vi "Autonomous Independent.vi"() -> ()   [LabVIEW 2013]
doc: "This VI is called when autonomous begins, and will automatically be terminated when autonomous ends. You can carry out timed or sensor driven robot movement independently without needing to return to the caller."
uses:
  Robot Global Data.vi
  <vilib>/Rock Robotics/WPI/RobotDrive/WPI_RobotDriveArcadeDrive_Standard(NoSaturation).vi
  <vilib>/Rock Robotics/WPI/RobotDrive/WPI_RobotDriveGetSetRefNum.vi
  <vilib>/Rock Robotics/WPI/Joystick/WPI_JoystickGetSetRefNum.vi
panel:
  out "Current Movement, for debugging":T1 {"Y Joystick Value" scale=1.0..-1.0; "X Joystick Value" scale=-1.0..1.0}
  in  "Array of robot movements":T2(array[cluster]) {"Y Joystick Value" scale=1.0..-1.0; "X Joystick Value" scale=-1.0..1.0}
  # "Be sure to right-click and choose Data Operations>>Make Current Value default if you want to save the array values with the VI"
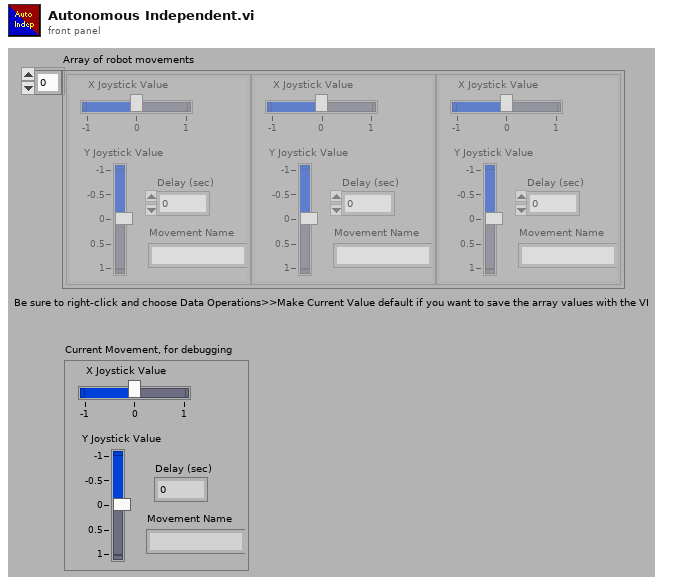
[diagram p1: front panel]
types:
  T1 = cluster{"X Joystick Value":dbl, "Y Joystick Value":dbl, "Delay (sec)":dbl, "Movement Name":string}
  T2 = cluster{"X Joystick Value":dbl, "Y Joystick Value":dbl, "Delay (sec)":dbl, "Movement Name":string}[]
  T3 = typedef "WPI_JoystickDevRef.ctl" = cluster{"Device":T4}
  T4 = typedef "WPI_JoystickDeviceEnum.ctl" = enum16{"USB 1", "USB 2", "USB 3", "USB 4", "Kinect 1", "Kinect 2"}
  T5 = cluster{"axis 1 (x)":dbl, "axis 2 (y)":dbl, "axis 3 (throttle)":dbl, "axis 4":dbl, "axis 5":dbl, "axis 6":dbl}
  T6 = typedef "WPI_RobotDriveDevRef.ctl" = cluster{"DevStatus":errorcluster, "Motors[]":T7[], "Square Inputs":bool, "Max Output":dbl, "Isochronous":bool}
  T7 = typedef "WPI_MotorControlDeviceRef.ctl" = cluster{"DeviceStatus":errorcluster, "Type":enum16{"PWM", "CAN"}, "PWM":cluster{"Digital Module":T8, "PWM Channel":T9, "DeadBand":T10}, "CAN":cluster{"Device Number":u8, "Control Mode":T11, "Semaphore":T12, "Max Vout":dbl}, "Invert":bool, "TransformRef":T13, "InvTransformRef":T13}
  T8 = typedef "FPGA_TypedefDigitalModule.ctl" = enum16{"Digital Module 1", "Digital Module 2"}
  T9 = typedef "FPGA_DIOPWMChannel.ctl" = enum8{"PWM 1", "PWM 2", "PWM 3", "PWM 4", "PWM 5", "PWM 6", "PWM 7", "PWM 8", "PWM 9", "PWM 10", "Invalid"}
  T10 = typedef "WPI_PWMDeadband.ctl" = cluster{"Name":string, "maxPositivePwm":i32, "minPositivePwm":i32, "centerPwm":i32, "maxNegativePwm":i32, "minNegativePwm":i32, "angularRange":u16}
  T11 = typedef "WPI_CANJaguar_ControlMode.ctl" = enum8{"Percent VBus", "Current", "Speed", "Position", "Voltage"}
  T12 = typedef "Semaphore RefNum" = refnum<k1>
  T13 = typedef "WPI_PWMTransform_ConPane.ctl" = refnum<vi>
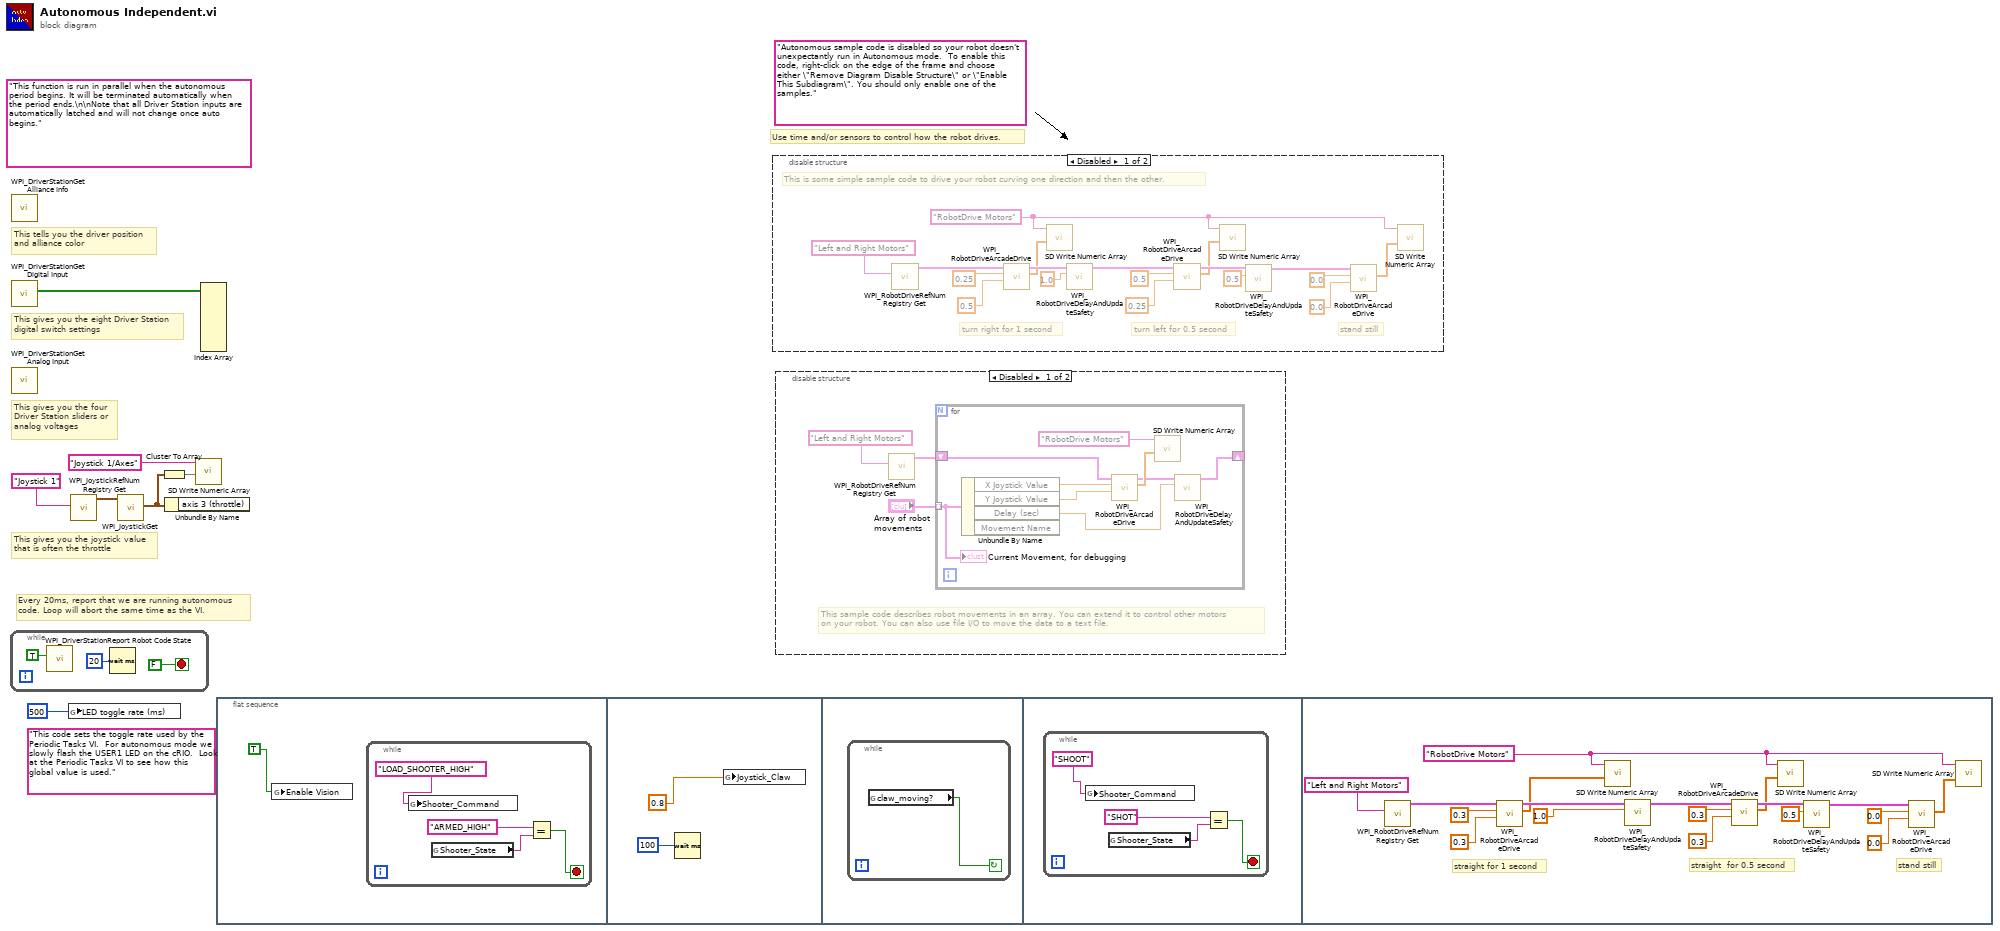
[diagram p0: block diagram]
diagram:
  (unwired) "This code sets the toggle rate used by the Periodic Tasks VI.  For autonomous mode we slowly flash the USER1 LED on the cRIO.  Look at the Periodic Tasks VI to see how this global value is used."
  (unwired) "Autonomous sample code is disabled so your robot doesn't unexpectantly run in Autonomous mode.  To enable this code, right-click on the edge of the frame and choose either \"Remove Diagram Disable Structure\" or \"Enable This Subdiagram\". You should only enable one of the samples."
  (unwired) "This function is run in parallel when the autonomous period begins. It will be terminated automatically when the period ends.\n\nNote that all Driver Station inputs are automatically latched and will not change once auto begins."
  # "Every 20ms, report that we are running autonomous\ncode. Loop will abort the same time as the VI."
  # "This gives you the joystick value\nthat is often the throttle"
  # "Use time and/or sensors to control how the robot drives."
  # "This tells you the driver position\nand alliance color"
  # "This gives you the eight Driver Station\ndigital switch settings"
  # "This gives you the four\nDriver Station sliders or\nanalog voltages"
  n1 = while {
    stop <- FALSE stop-if-true
    n2 = call <vilib>:"WPI_DriverStationReport Robot Code State.vi"("Autonomous"=TRUE) -> ()  [unwired: 10 in, 1 out]
    n3 = Wait (ms)(milliseconds to wait=u32 20) -> ()  [unwired: 1 out]
  }
  n4 = call <vilib>:"WPI_DriverStationGet Alliance Info.vi"() -> ()  [unwired: 12 out]
  n5 = call <vilib>:"WPI_DriverStationGet Digital Input.vi"() -> ("Driver Station Digital Input (1-8)"=w7:bool[])  [unwired: 11 out]
  n6 = call <vilib>:"WPI_DriverStationGet Analog Input.vi"() -> ()  [unwired: 12 out]
  n7 = global write "Robot Global Data.vi" "LED toggle rate (ms)"(u32 500 ("LED ms toggle rate")) -> ()
  n8 = call <vilib>:"WPI_JoystickRefNum Registry Get.vi"("refnum name"="Joystick 1") -> ("JoystickDevRef"=w5:T3)  [unwired: 1 in, 9 out]
  n9 = call <vilib>:"WPI_JoystickGet.vi"("JoystickDevRef"=w5) -> ("Axes"=w2:T5)  [unwired: 1 in, 5 out]
  n10 = Cluster To Array(cluster=w2) -> (array=w3:dbl[])
  n11 = Unbundle By Name(w2) -> ()  [unwired: 1 out]
  n12 = call <vilib>:"SD Write Numeric Array.vi"("Numeric Array"=w3, "Name"="Joystick 1/Axes") -> ()  [unwired: 8 in, 2 out]
  n13 = Index Array(array=w7) -> ()  [unwired: 8 in, 8 out]
  n14 = flat-sequence {
    frame #0 {
      n15 = global write "Robot Global Data.vi" "Enable Vision"(TRUE) -> ()
      n16 = while {
        stop <- w12 stop-if-true
        n17 = global write "Robot Global Data.vi" "Shooter_Command"("LOAD_SHOOTER_HIGH") -> ()
        n18 = global read "Robot Global Data.vi" "Shooter_State"() -> (w14:string)
        n19 = Equal?(x="ARMED_HIGH", y=w14) -> (x = y?=w12:bool)
      }
    }
    frame #1 {
      n20 = Wait (ms)(milliseconds to wait=100) -> ()  [unwired: 1 out]
      n21 = global write "Robot Global Data.vi" "Joystick_Claw"(0.8) -> ()
    }
    frame #2 {
      n22 = while {
        stop <- w18 continue-if-true
        n23 = global read "Robot Global Data.vi" "claw_moving?"() -> (w18:bool)
      }
    }
    frame #3 {
      n24 = while {
        stop <- w19 stop-if-true
        n25 = global write "Robot Global Data.vi" "Shooter_Command"("SHOOT") -> ()
        n26 = global read "Robot Global Data.vi" "Shooter_State"() -> (w21:string)
        n27 = Equal?(x="SHOT", y=w21) -> (x = y?=w19:bool)
      }
    }
    frame #4 {
      w23 = "RobotDrive Motors" ("Name")
      # "stand still"
      # "straight  for 0.5 second"
      # "straight for 1 second"
      n28 = call <vilib>:"WPI_RobotDriveRefNum Registry Get.vi"("refnum name"="Left and Right Motors") -> ("RobotDriveDevRef"=w27:T6)  [unwired: 1 in, 9 out]
      n29 = call-poly <vilib>:"WPI_RobotDriveArcadeDrive.vi"("Y axis value"=0.3 ("X axis value"), "X axis value"=0.3, "RobotDriveDevRef"=w27) -> ("Motor Values"=w26:dbl[], "RobotDriveDevRef"=w34:T6)  [unwired: 1 in, 6 out]
      n30 = call <vilib>:"SD Write Numeric Array.vi"("Numeric Array"=w26, "Name"=w23) -> ()  [unwired: 8 in, 2 out]
      n31 = call <vilib>:"WPI_RobotDriveDelayAndUpdateSafety.vi"("Delay (s)"=1.0, "RobotDriveDevRef"=w34) -> ("RobotDriveDevRef 2"=w33:T6)  [unwired: 8 in, 1 out]
      n32 = call-poly <vilib>:"WPI_RobotDriveArcadeDrive.vi"("Y axis value"=0.3 ("X axis value"), "X axis value"=0.3, "RobotDriveDevRef"=w33) -> ("Motor Values"=w25:dbl[], "RobotDriveDevRef"=w32:T6)  [unwired: 1 in, 6 out]
      n33 = call <vilib>:"SD Write Numeric Array.vi"("Numeric Array"=w25, "Name"=w23) -> ()  [unwired: 8 in, 2 out]
      n34 = call <vilib>:"WPI_RobotDriveDelayAndUpdateSafety.vi"("Delay (s)"=0.5, "RobotDriveDevRef"=w32) -> ("RobotDriveDevRef 2"=w31:T6)  [unwired: 8 in, 1 out]
      n35 = call-poly <vilib>:"WPI_RobotDriveArcadeDrive.vi"("Y axis value"=0.0 ("X axis value"), "X axis value"=0.0, "RobotDriveDevRef"=w31) -> ("Motor Values"=w24:dbl[])  [unwired: 1 in, 7 out]
      n36 = call <vilib>:"SD Write Numeric Array.vi"("Numeric Array"=w24, "Name"=w23) -> ()  [unwired: 8 in, 2 out]
    }
  }
  n37 = disable-structure shown="Disabled" {
    frame Disabled {
      w41 = "RobotDrive Motors" ("Name")
      # "This is some simple sample code to drive your robot curving one direction and then the other."
      # "stand still"
      # "turn left for 0.5 second"
      # "turn right for 1 second"
      n38 = call <vilib>:"WPI_RobotDriveRefNum Registry Get.vi"("refnum name"="Left and Right Motors") -> ("RobotDriveDevRef"=w45:T6)  [unwired: 1 in, 9 out]
      n39 = call-poly <vilib>:"WPI_RobotDriveArcadeDrive.vi"("Y axis value"=0.5 ("X axis value"), "X axis value"=0.25, "RobotDriveDevRef"=w45) -> ("Motor Values"=w44:dbl[], "RobotDriveDevRef"=w52:T6)  [unwired: 1 in, 6 out]
      n40 = call <vilib>:"SD Write Numeric Array.vi"("Numeric Array"=w44, "Name"=w41) -> ()  [unwired: 8 in, 2 out]
      n41 = call <vilib>:"WPI_RobotDriveDelayAndUpdateSafety.vi"("Delay (s)"=1.0, "RobotDriveDevRef"=w52) -> ("RobotDriveDevRef 2"=w51:T6)  [unwired: 8 in, 1 out]
      n42 = call-poly <vilib>:"WPI_RobotDriveArcadeDrive.vi"("Y axis value"=0.25 ("X axis value"), "X axis value"=0.5, "RobotDriveDevRef"=w51) -> ("Motor Values"=w43:dbl[], "RobotDriveDevRef"=w50:T6)  [unwired: 1 in, 6 out]
      n43 = call <vilib>:"SD Write Numeric Array.vi"("Numeric Array"=w43, "Name"=w41) -> ()  [unwired: 8 in, 2 out]
      n44 = call <vilib>:"WPI_RobotDriveDelayAndUpdateSafety.vi"("Delay (s)"=0.5, "RobotDriveDevRef"=w50) -> ("RobotDriveDevRef 2"=w49:T6)  [unwired: 8 in, 1 out]
      n45 = call-poly <vilib>:"WPI_RobotDriveArcadeDrive.vi"("Y axis value"=0.0 ("X axis value"), "X axis value"=0.0, "RobotDriveDevRef"=w49) -> ("Motor Values"=w42:dbl[])  [unwired: 1 in, 7 out]
      n46 = call <vilib>:"SD Write Numeric Array.vi"("Numeric Array"=w42, "Name"=w41) -> ()  [unwired: 8 in, 2 out]
    }
    frame Enabled {
    }
  }
  n47 = disable-structure shown="Disabled" {
    frame Disabled {
      # "This sample code describes robot movements in an array. You can extend it to control other motors\non your robot. You can also use file I/O to move the data to a text file."
      n48 = call <vilib>:"WPI_RobotDriveRefNum Registry Get.vi"("refnum name"="Left and Right Motors") -> ("RobotDriveDevRef"=w60:T6)  [unwired: 1 in, 9 out]
      n49 = for {
        shift-right: [w66] -> _
        shift-left: w60 -> [w67]
        tunnel: "Array of robot movements" -> [w62] mode=indexing
        n50 = Unbundle By Name(w62) -> ("X Joystick Value"=w65:dbl, "Y Joystick Value"=w64:dbl, "Delay (sec)"=w63:dbl)  [unwired: 1 out]
        n51 = call-poly <vilib>:"WPI_RobotDriveArcadeDrive.vi"("Y axis value"=w64, "X axis value"=w65, "RobotDriveDevRef"=w67) -> ("Motor Values"=w69:dbl[], "RobotDriveDevRef"=w68:T6)  [unwired: 1 in, 6 out]
        n52 = call <vilib>:"SD Write Numeric Array.vi"("Numeric Array"=w69, "Name"="RobotDrive Motors") -> ()  [unwired: 8 in, 2 out]
        n53 = call <vilib>:"WPI_RobotDriveDelayAndUpdateSafety.vi"("Delay (s)"=w63, "RobotDriveDevRef"=w68) -> ("RobotDriveDevRef 2"=w66:T6)  [unwired: 8 in, 1 out]
        "Current Movement, for debugging" <- w62
      }
    }
    frame Enabled {
    }
  }
